vi "welcome.vi"   [LabVIEW 2018]
uses:
  user32.dll
types:
  T1 = enum32{"Invalid", "Standard", "Closed", "Hidden", "Minimized", "Maximized"}
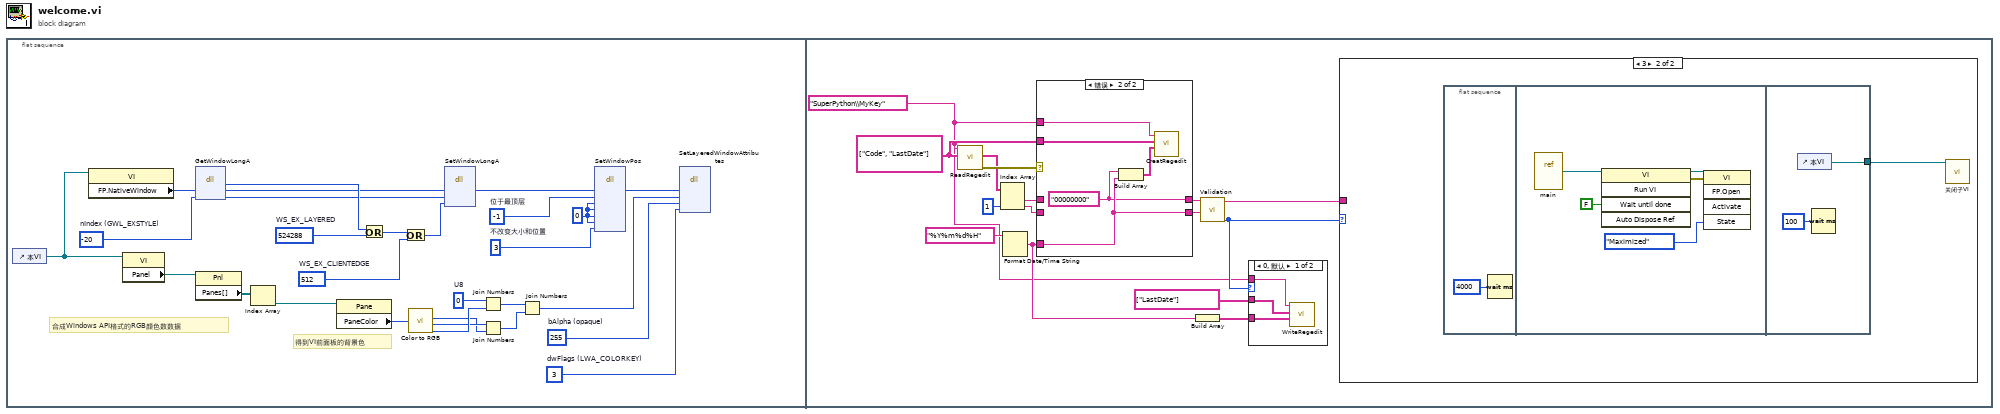
[diagram p0: block diagram]
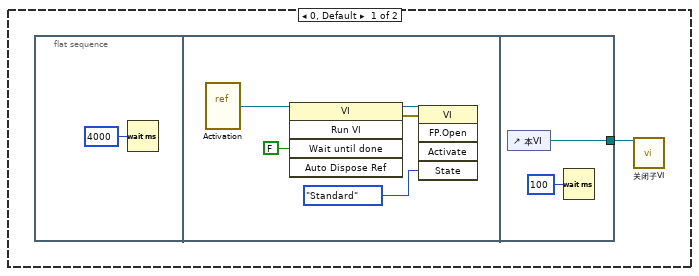
[diagram p2: hidden frame]
diagram:
  n1 = flat-sequence {
    frame #0 {
      w25 = 512  # WS_EX_CLIENTEDGE
      w21 = 3  # 不改变大小和位置
      w24 = 0 ("nIndex")
      w20 = -1  # 位于最顶层
      w2 = 255  # bAlpha (opaque)
      w1 = 3  # dwFlags (LWA_COLORKEY)
      w9 = u8 0  # U8
      w17 = 524288  # WS_EX_LAYERED
      w18 = -20  # nIndex (GWL_EXSTYLE)
      # "合成Windows API格式的RGB颜色数数据"
      # "得到VI前面板的背景色"
      n2 = control-ref of="本VI"() -> (w28:refnum<vi>)
      n3 = property class="VI"(reference=w28) -> ("FP.NativeWindow"=w19:u64)  [unwired: 1 in, 2 out]
      n4 = property class="VI"(reference=w28) -> ("Panel"=w4:refnum<vi>)  [unwired: 1 in, 2 out]
      n5 = dll-call lib="user32.dll" fn="GetWindowLongA"("handle"=w19, "nIndex"=w18) -> ("返回类型"=w16:i32, "handle"=w15:i32, "nIndex"=w14:i32)  [unwired: 3 in, 2 out]
      n6 = property class="Pnl"(reference=w4) -> ("Panes[]"=w5:refnum<vi>[])  [unwired: 1 in, 2 out]
      n7 = Index Array(array=w5) -> (element=w6:refnum<vi>)  [unwired: 1 in]
      n8 = property class="Pane"(reference=w6) -> ("PaneColor"=w10:u32)  [unwired: 1 in, 2 out]
      n9 = Or(x=w16, y=w17) -> (x .or. y?=w26:i32)
      n10 = Or(x=w26, y=w25) -> (x .or. y?=w27:i32)
      n11 = call <vilib>:"Color to RGB.vi"("Color"=w10) -> ("R"=w11:u8, "G"=w12:u8, "B"=w13:u8)  [unwired: 1 out]
      n12 = dll-call lib="USER32.DLL" fn="SetWindowLongA" label="SetWindowLong"("handle"=w15, "nIndex"=w14, "dwNewLong"=w27) -> ("handle"=w22:i32)  [unwired: 5 in, 3 out]
      n13 = Join Numbers(hi=w9, lo=w13) -> ((hi.lo)=w8:u16)
      n14 = Join Numbers(hi=w12, lo=w11) -> ((hi.lo)=w7:u16)
      n15 = Join Numbers(hi=w8, lo=w7) -> ((hi.lo)=w3:u32)
      n16 = dll-call lib="USER32.DLL" fn="SetWindowPos"("hWnd"=w22, "hWndInsertAfter"=w20, "x"=w24, "y"=w24, "cx"=w24, "cy"=w24, "wFlags"=w21) -> ("hWnd"=w23:i32)  [unwired: 9 in, 3 out]
      n17 = dll-call lib="USER32.DLL" fn="SetLayeredWindowAttributes" label="SetLayerdWindowAttributs"("handle"=w23, "crkey"=w3, "bAlpha"=w2, "dwFlags"=w1) -> ()  [unwired: 7 in, 3 out]
    }
    frame #1 {
      w29 = "SuperPython\\MyKey" ("subkey")
      w36 = string[] ["Code", "LastDate"]
      n18 = call "ReadRegedit.vi"("名称"=w36, "subkey"=w29) -> ("error out"=w40:errorcluster, "值"=w35:string[])  [unwired: 8 in]
      n19 = Index Array(array=w35, index #2=1 ("索引")) -> (element #1=w38:string, element #2=w37:string)  [unwired: 1 in]
      n20 = Format Date/Time String(time format string (%c)="%Y%m%d%H" ("时间格式字符串(%c)")) -> (date/time string=w33:string)  [unwired: 2 in]
      n21 = case shown="错误" w40 {
        tunnel: w38 -> [w65 _]
        tunnel: [w65 w69] -> w43
        tunnel: w37 -> [w66 _]
        tunnel: [w66 w70] -> w42
        tunnel: w33 -> [_ w70]
        tunnel: w36 -> [_ w71]
        tunnel: w29 -> [_ w67]
        frame No Error {
        }
        frame Error {
          w69 = "00000000" ("String/Binary data")
          n22 = Build Array(w69, w70) -> (w68:string[])
          n23 = call "CreatRegedit.vi"("值"=w68, "名称"=w71, "subkey"=w67) -> ()  [unwired: 8 in, 1 out]
        }
      }
      n24 = Build Array(w33) -> (w32:string[])
      n25 = call "Validation.vi"("Date"=w42, "Password"=w43) -> ("激活状态"=w31:i32, "提示符"=w30:string)  [unwired: 7 in, 1 out]
      n26 = case shown="0, 默认" w31 {
        tunnel: string[] ["LastDate"] -> [w64 _]
        tunnel: w32 -> [w63 _]
        tunnel: w29 -> [w62 _]
        frame 0, Default {
          n27 = call "WriteRegedit.vi"("值"=w63, "名称"=w64, "subkey"=w62) -> ()  [unwired: 8 in, 1 out]
        }
        frame 2 {
        }
      }
      n28 = case shown="3" w31 {
        tunnel: w30 -> [_ _]
        frame 0, Default {
          n29 = flat-sequence {
            tunnel: [w52] -> w44
            frame #0 {
              n30 = Wait (ms)(milliseconds to wait=u32 4000 ("等待时间（毫秒）")) -> ()  [unwired: 1 out]
            }
            frame #1 {
              n31 = vi-ref "Activation.vi"() -> (w46:refnum<vi>)
              n32 = invoke class="VI" method="Run VI"(reference=w46, "Wait until done"=FALSE ("结束前等待")) -> (reference out=w49:refnum<vi>, error out=w50:errorcluster)  [unwired: 3 in, 3 out]
              n33 = invoke class="VI" method="FP.Open"(reference=w49, error in=w50, "State"=T1."Standard" ("状态")) -> ()  [unwired: 2 in, 5 out]
            }
            frame #2 {
              n34 = control-ref of="本VI"() -> (w52:refnum<vi>)
              n35 = Wait (ms)(milliseconds to wait=u32 100 ("等待时间（毫秒）")) -> ()  [unwired: 1 out]
            }
          }
          n36 = call "关闭子VI.vi"("引用"=w44) -> ()  [unwired: 9 in, 2 out]
        }
        frame 3 {
          n37 = flat-sequence {
            tunnel: [w60] -> w53
            frame #0 {
              n38 = Wait (ms)(milliseconds to wait=u32 4000 ("等待时间（毫秒）")) -> ()  [unwired: 1 out]
            }
            frame #1 {
              n39 = vi-ref "main.vi"() -> (w55:refnum<vi>)
              n40 = invoke class="VI" method="Run VI"(reference=w55, "Wait until done"=FALSE ("结束前等待")) -> (reference out=w58:refnum<vi>, error out=w59:errorcluster)  [unwired: 3 in, 3 out]
              n41 = invoke class="VI" method="FP.Open"(reference=w58, error in=w59, "State"=T1."Maximized" ("状态")) -> ()  [unwired: 2 in, 5 out]
            }
            frame #2 {
              n42 = control-ref of="本VI"() -> (w60:refnum<vi>)
              n43 = Wait (ms)(milliseconds to wait=u32 100 ("等待时间（毫秒）")) -> ()  [unwired: 1 out]
            }
          }
          n44 = call "关闭子VI.vi"("引用"=w53) -> ()  [unwired: 9 in, 2 out]
        }
      }
    }
  }
